vi "button_main_02.vi"() -> ()   [LabVIEW 2023]
panel:
  out "Start_aux":bool
  in  "Start":bool
  in  "Stop Button":bool
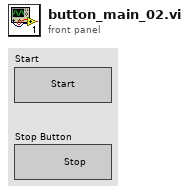
[diagram p1: front panel]
types:
  T1 = enum32{"Bad", "Idle", "Run top level", "Running"}
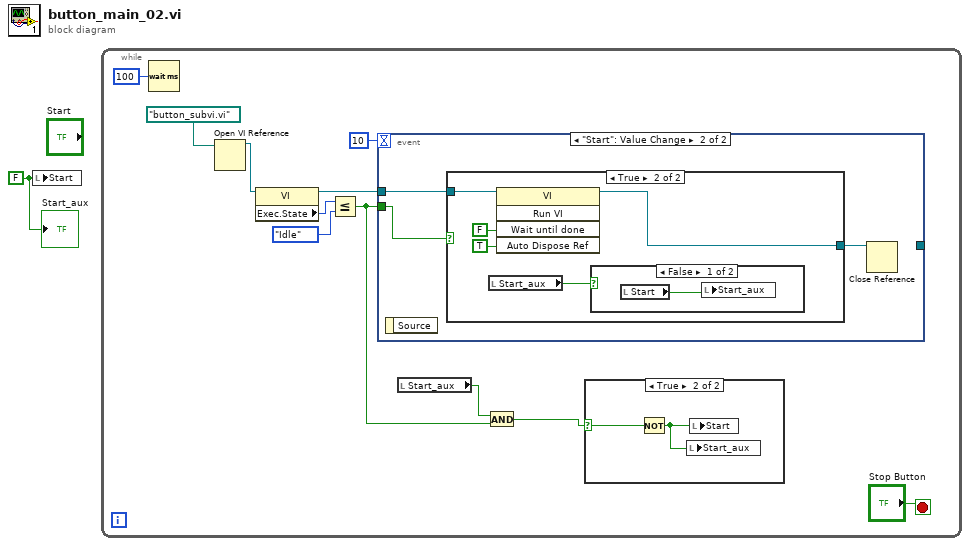
[diagram p0: block diagram]
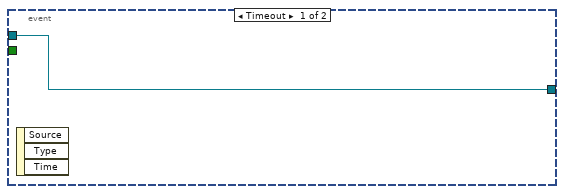
[diagram p2: hidden frame]
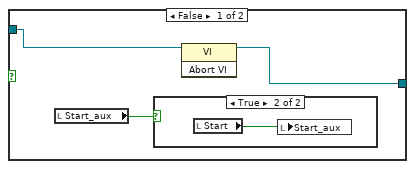
[diagram p3: hidden frame]
diagram:
  w1 = FALSE ("Start")
  n1 = local write "Start"(w1) -> ()
  n2 = while {
    stop <- "Stop Button" stop-if-true
    n3 = Wait (ms)(milliseconds to wait=u32 100) -> ()  [unwired: 1 out]
    n4 = Open VI Reference(vi path=path "button_subvi.vi") -> (vi reference=w2:refnum<vi>)  [unwired: 5 in, 1 out]
    n5 = property class="VI"(reference=w2) -> (reference out=w5:refnum<vi>, "Exec.State"=w6:T1)  [unwired: 1 in, 1 out]
    n6 = Less Or Equal?(x=w6, y=T1."Idle" ("Execution:State")) -> (x <= y?=w4:bool)
    n7 = event shown="[1] \"Start\": Value Change" {
      selector: _ -> [_ _]
      dyn-events: _ -> [_ _]
      timeout: 10 -> [_ _]
      tunnel: w5 -> [w13 w15]
      tunnel: w4 -> [_ w16]
      tunnel: [w13 _] -> _
      event Timeout {
        n8 = event-data() -> ()  [unwired: 1 in, 3 out]
      }
      event "Start": Value Change {
        n9 = event-data() -> ()  [unwired: 1 in, 1 out]
        n10 = case shown="True" w16 {
          tunnel: w15 -> [w19 w23]
          tunnel: [w18 w22] -> w14
          frame False {
            n11 = local read "Start_aux"() -> (w17:bool)
            n12 = case shown="True" w17 {
              frame False {
              }
              frame True {
                n13 = local read "Start"() -> (w20:bool)
                n14 = local write "Start_aux"(w20) -> ()
              }
            }
            n15 = invoke class="VI" method="Abort VI"(reference=w19) -> (reference out=w18:refnum<vi>)  [unwired: 2 in, 2 out]
          }
          frame True {
            n16 = local read "Start_aux"() -> (w21:bool)
            n17 = invoke class="VI" method="Run VI"(reference=w23, "Wait until done"=FALSE ("Wait Until Done"), "Auto Dispose Ref"=TRUE ("Auto Dispose Reference")) -> (reference out=w22:refnum<vi>)  [unwired: 2 in, 4 out]
            n18 = case shown="False" w21 {
              frame False {
                n19 = local read "Start"() -> (w26:bool)
                n20 = local write "Start_aux"(w26) -> ()
              }
              frame True {
              }
            }
          }
        }
        n21 = Close Reference(reference=w14) -> ()  [unwired: 1 in, 1 out]
      }
    }
    n22 = local read "Start_aux"() -> (w8:bool)
    n23 = And(x=w8, y=w4) -> (x .and. y?=w9:bool)
    n24 = case shown="True" w9 {
      selector: w9 -> [_ w28]
      frame False {
      }
      frame True {
        n25 = Not(x=w28) -> (.not. x?=w27:bool)
        n26 = local write "Start_aux"(w27) -> ()
        n27 = local write "Start"(w27) -> ()
      }
    }
  }
  "Start_aux" <- w1
